vi "CVT Double GetIndex.vi"(8 "error in (no error)":errorcluster, 11 "Tag Name":string) -> (0 "error out":errorcluster, 3 "Index":i32)   [LabVIEW 2020, in "Current Value Table(Rebuild).lvlib"]
uses:
  Current Value Table(Rebuild).lvlib
  DataTypes/Double_Get Index.vi
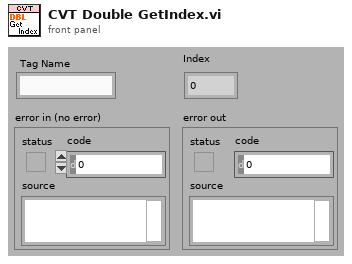
[diagram p1: front panel]
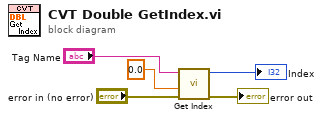
[diagram p0: block diagram]
diagram:
  n1 = call-poly "Get Index.vi"("error in (no error)"="error in (no error)", "Default"=0.0 ("Data Type"), "Tag Name"="Tag Name") -> ("error out"=→"error out":errorcluster, "Index"=→"Index":i32)  [unwired: 7 in]
